vi "comm buffer.vi"(8 "error in (no error)":errorcluster, 9 "Out Queue Size":u32, 10 "In Queue Size":u32, 11 "Comm Handle":u64) -> (0 "error out":errorcluster, 3 "dup Comm Handle":u64)   [LabVIEW 2021, in "lvserial.lvlib"]
doc: "The SetupComm function initializes the communications parameters for a specified communications device. \nThe GetCommState function retrieves the current control settings for a specified communications device."
uses:
  lvserial.lvlib
  lvserial.dll
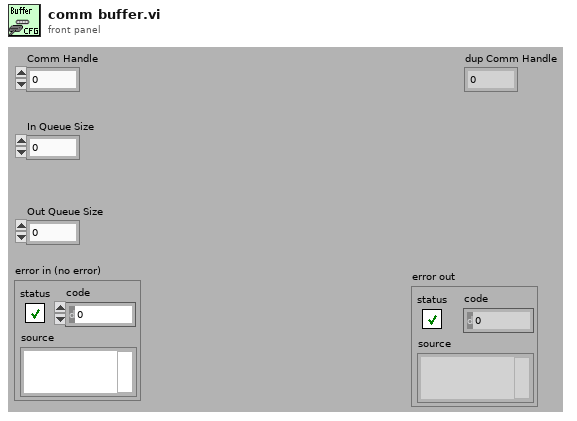
[diagram p1: front panel]
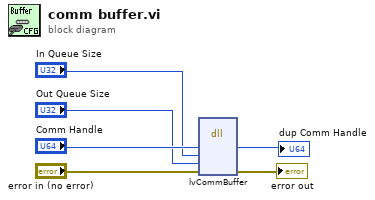
[diagram p0: block diagram]
diagram:
  n1 = dll-call lib="lvserial.dll" fn="lvCommBuffer"("hComm"="Comm Handle", "ulInQueueSize"="In Queue Size", "ulInQueueSize"="Out Queue Size", "error"="error in (no error)") -> ("hComm"=→"dup Comm Handle":u64, "error"=→"error out":errorcluster)  [unwired: 5 in, 3 out]
